vi "PRL PMU Status Private.vi"(10 "PMU Status In":T1(array[cluster]), 11 "Read(T)/Write(F)":bool=TRUE) -> (3 "PMU Status Out":T1(array[cluster]))   [LabVIEW 2017, in "PMU Recorder Light.lvlib"]
uses:
  PMU Recorder Light.lvlib
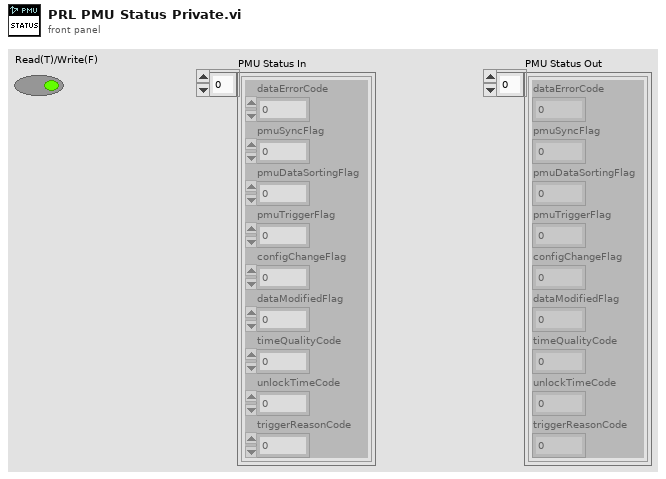
[diagram p1: front panel]
types:
  T1 = cluster{"dataErrorCode":u8, "pmuSyncFlag":u8, "pmuDataSortingFlag":u8, "pmuTriggerFlag":u8, "configChangeFlag":u8, "dataModifiedFlag":u8, "timeQualityCode":u8, "unlockTimeCode":u8, "triggerReasonCode":u8}[]
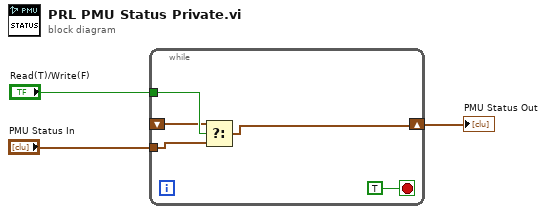
[diagram p0: block diagram]
diagram:
  n1 = while {
    tunnel: "PMU Status In" -> [w5]
    shift-right: [w6] -> w1
    shift-left: _ -> [w7]
    tunnel: "Read(T)/Write(F)" -> [w8]
    stop <- TRUE stop-if-true
    n2 = Select(t=w7, s=w8, f=w5) -> (s? t:f=w6:T1)
  }
  "PMU Status Out" <- w1
